vi "Motion Profile Generater-Demo.vi"(0 "Max Speed (rotations/sec)":dbl, 5 "Max Acceleration (rotations/sec^2)":dbl, 7 "Max Jerk (rotations/sec^3)":dbl, 9 "Rotations to Travel":dbl, 11 "Motion Profile Control Frame Rate":dbl) -> (4 "Position rotations":dbl[](array[numeric]), 6 "velocity rotations/sec":dbl[](array[numeric]), 8 "acceleration rotations/sec^2":dbl[](array[numeric]))   [LabVIEW 2015]
panel:
  out "Final Position":dbl
  out "XY Graph":cluster{dbl[], dbl[]}[](graph)
  # "NOTE: this method doesn't work (unknown reasons) when we don't reach max acceleration or\n we don't reach max speed"
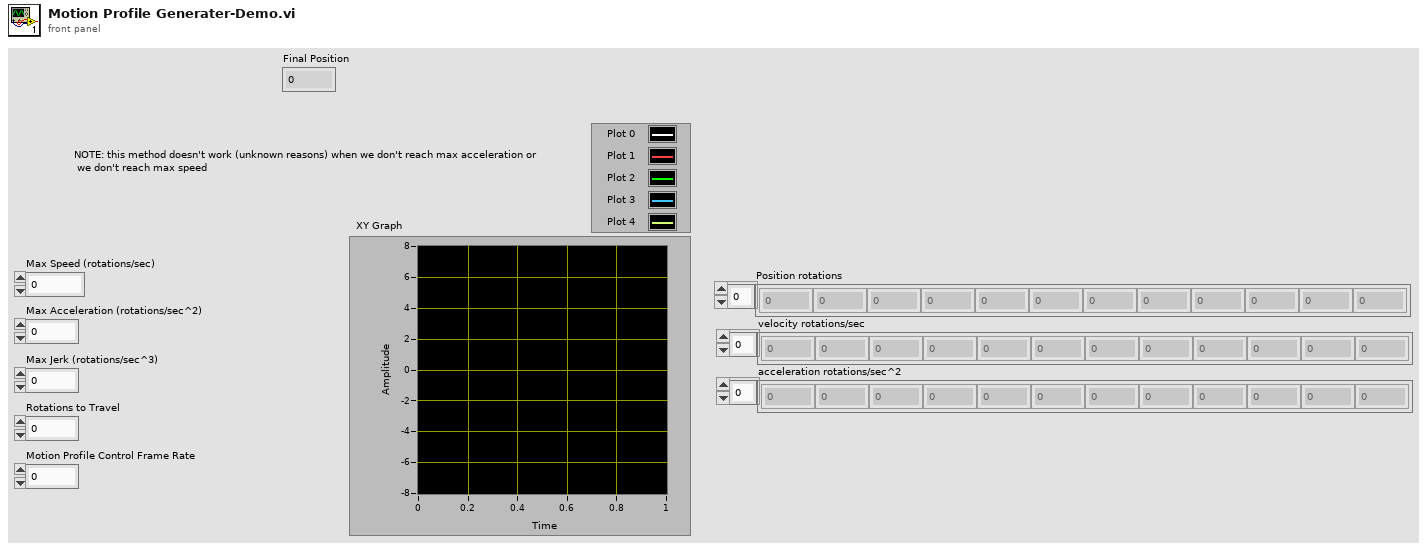
[diagram p1: front panel]
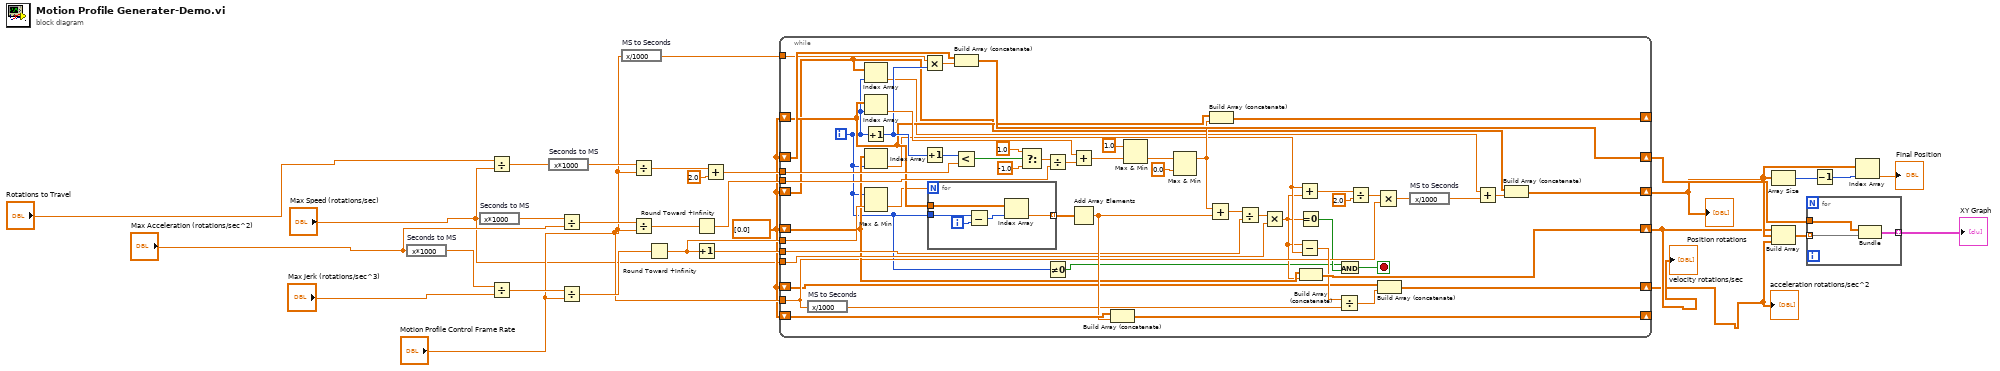
[diagram p0: block diagram]
diagram:
  w14 = dbl[] [0.0]
  n1 = expression code="x*1000" "Seconds to MS"("Max Acceleration (rotations/sec^2)") -> (w29:dbl)
  n2 = expression code="x*1000" "Seconds to MS"("Max Speed (rotations/sec)") -> (w28:dbl)
  n3 = Divide(x="Rotations to Travel", y="Max Speed (rotations/sec)") -> (x/y=w27:dbl)
  n4 = Divide(x=w29, y="Max Jerk (rotations/sec^3)") -> (x/y=w19:dbl)
  n5 = expression code="x*1000" "Seconds to MS"(w27) -> (w26:dbl)
  n6 = Divide(x=w28, y="Max Acceleration (rotations/sec^2)") -> (x/y=w22:dbl)
  n7 = Divide(x=w19, y="Motion Profile Control Frame Rate") -> (x/y=w18:dbl)
  n8 = expression code="x/1000" "MS to Seconds"("Motion Profile Control Frame Rate") -> (w30:dbl)
  n9 = Divide(x=w26, y="Motion Profile Control Frame Rate") -> (x/y=w25:dbl)
  n10 = Divide(x=w22, y="Motion Profile Control Frame Rate") -> (x/y=w21:dbl)
  n11 = Round Toward +Infinity(x=w18) -> (ceil(x): smallest int >= x=w17:dbl)
  n12 = Round Toward +Infinity(x=w21) -> (ceil(x): smallest int >= x=w20:dbl)
  n13 = Increment(x=w17) -> (x+1=w16:dbl)
  n14 = Add(x=w25, y=2.0) -> (x+y=w23:dbl)
  n15 = while {
    shift-right: [w83] -> w12
    shift-left: w14 -> [w84]
    tunnel: w30 -> [w82]
    tunnel: w23 -> [w80]
    shift-right: [w66] -> _
    shift-left: w14 -> [w65]
    tunnel: w20 -> [w72]
    tunnel: w17 -> [w63]
    shift-right: [w60] -> _
    shift-left: w14 -> [w61]
    tunnel: w16 -> [w56]
    tunnel: "Max Speed (rotations/sec)" -> [w54]
    shift-right: [w53] -> w2
    shift-left: w14 -> [w51]
    shift-right: [w52] -> w3
    shift-left: w14 -> [w45]
    tunnel: "Motion Profile Control Frame Rate" -> [w39]
    shift-right: [w37] -> w1
    shift-left: w14 -> [w36]
    i -> [w35]
    stop <- w31 stop-if-true
    n16 = expression code="x/1000" "MS to Seconds"(w39) -> (w40:dbl)
    n17 = Index Array(array=w45, index=w35) -> (element=w44:dbl)
    n18 = Index Array(array=w65, index=w35) -> (element=w70:dbl)
    n19 = Increment(x=w35) -> (x+1=w68:i32)
    n20 = Index Array(array=w51, index=w35) -> (element=w42:dbl)
    n21 = Max & Min(x=w35, y=w63) -> (min(x,y)=w62:dbl)  [unwired: 1 out]
    n22 = Multiply(x=w82, y=w68) -> (x*y=w81:dbl)
    n23 = Increment(x=w68) -> (x+1=w69:i32)
    n24 = for {
      N: w62 -> [_]
      tunnel: w35 -> [w88]
      tunnel: w65 -> [w86]
      tunnel: [w85] -> w64 mode=indexing
      i -> [w89]
      n25 = Subtract(x=w88, y=w89) -> (x-y=w87:i32)
      n26 = Index Array(array=w86, index=w87) -> (element=w85:dbl)
    }
    n27 = Less?(x=w69, y=w80) -> (x < y?=w76:bool)
    n28 = Build Array (concatenate)(w84, w81) -> (w83:dbl[])
    n29 = Select(t=1.0, s=w76, f=-1.0) -> (s? t:f=w73:dbl)
    n30 = Divide(x=w73, y=w72) -> (x/y=w71:dbl)
    n31 = Not Equal To 0?(x=w35) -> (x != 0?=w32:bool)
    n32 = Add(x=w70, y=w71) -> (x+y=w67:dbl)
    n33 = Add Array Elements(numeric array=w64) -> (sum=w59:dbl)
    n34 = Build Array (concatenate)(w61, w59) -> (w60:dbl[])
    n35 = Max & Min(x=1.0, y=w67) -> (min(x,y)=w78:dbl)  [unwired: 1 out]
    n36 = Max & Min(x=w78, y=0.0) -> (max(x,y)=w58:dbl)  [unwired: 1 out]
    n37 = Add(x=w58, y=w59) -> (x+y=w57:dbl)
    n38 = Build Array (concatenate)(w65, w58) -> (w66:dbl[])
    n39 = Divide(x=w57, y=w56) -> (x/y=w55:dbl)
    n40 = Multiply(x=w55, y=w54) -> (x*y=w34:dbl)
    n41 = Add(x=w42, y=w34) -> (x+y=w50:dbl)
    n42 = Subtract(x=w34, y=w42) -> (x-y=w41:dbl)
    n43 = Equal To 0?(x=w34) -> (x = 0?=w33:bool)
    n44 = Build Array (concatenate)(w51, w34) -> (w53:dbl[])
    n45 = Divide(x=w41, y=w40) -> (x/y=w38:dbl)
    n46 = And(x=w32, y=w33) -> (x .and. y?=w31:bool)
    n47 = Divide(x=w50, y=2.0) -> (x/y=w48:dbl)
    n48 = Multiply(x=w48, y=w39) -> (x*y=w47:dbl)
    n49 = Build Array (concatenate)(w36, w38) -> (w37:dbl[])
    n50 = expression code="x/1000" "MS to Seconds"(w47) -> (w46:dbl)
    n51 = Add(x=w44, y=w46) -> (x+y=w43:dbl)
    n52 = Build Array (concatenate)(w45, w43) -> (w52:dbl[])
  }
  "velocity rotations/sec" <- w2
  "Position rotations" <- w3
  "acceleration rotations/sec^2" <- w1
  n53 = Array Size(array=w3) -> (size(s)=w10:i32)
  n54 = Build Array(w2, w3, w1) -> (w13:dbl[][])
  n55 = for {
    tunnel: w13 -> [w92] mode=indexing
    tunnel: w12 -> [w91]
    tunnel: [w90] -> w11 mode=indexing
    n56 = Bundle(w91, w92) -> (w90:cluster{dbl[], dbl[]})  [unwired: 1 in]
  }
  "XY Graph" <- w11
  n57 = Decrement(x=w10) -> (x-1=w9:i32)
  n58 = Index Array(array=w3, index=w9) -> (element=→"Final Position":dbl)
